vi "in_ensure monotonic.vi"(8 "X is monotonic":bool, 10 "Y":dbl[](array[numeric]), 11 "X":dbl[](array[numeric])) -> (2 "Y out":dbl[](array[numeric]), 3 "X out":dbl[](array[numeric]))   [LabVIEW 2010, in "NI_Gmath.lvlib"]
uses:
  NI_Gmath.lvlib
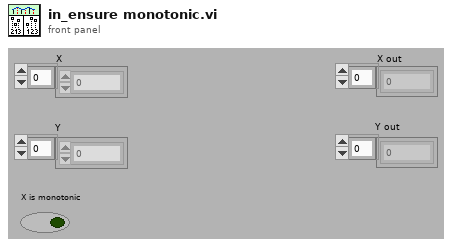
[diagram p1: front panel]
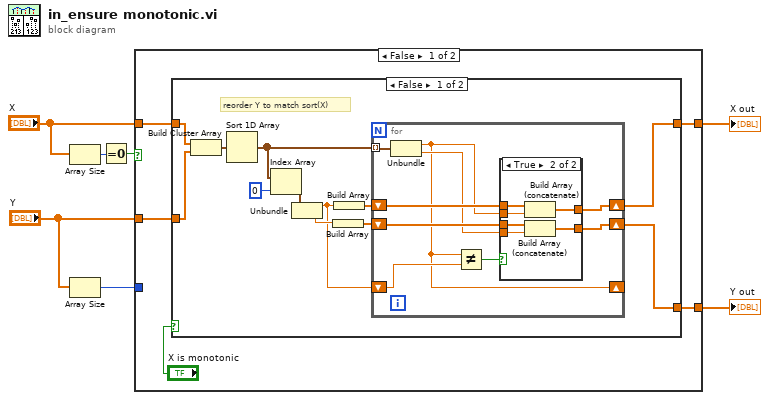
[diagram p0: block diagram]
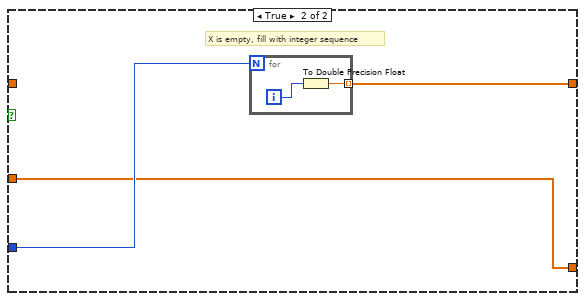
[diagram p4: hidden frame]
diagram:
  n1 = Array Size(array="X") -> (size(s)=w7:i32)
  n2 = Array Size(array="Y") -> (size(s)=w6:i32)
  n3 = Equal To 0?(x=w7) -> (x = 0?=w5:bool)
  n4 = case shown="False" w5 {
    tunnel: w6 -> [_ w46]
    tunnel: [w10 w44] -> w2
    tunnel: "X" -> [w12 _]
    tunnel: [w9 w45] -> w3
    tunnel: "Y" -> [w11 w44]
    frame False {
      n5 = case shown="False" "X is monotonic" {
        tunnel: w12 -> [w23 w42]
        tunnel: w11 -> [w22 w43]
        tunnel: [w13 w43] -> w10
        tunnel: [w14 w42] -> w9
        frame False {
          # "reorder Y to match sort(X)"
          n6 = Build Cluster Array(w23, w22) -> (w24:cluster{"Numeric":dbl, "Numeric":dbl}[])
          n7 = Sort 1D Array(array=w24) -> (sorted array=w21:cluster{"Numeric":dbl, "Numeric":dbl}[])
          n8 = Index Array(array=w21, index=0) -> (element=w19:cluster{"Numeric":dbl, "Numeric":dbl})
          n9 = Unbundle(w19) -> ("Numeric"=w15:dbl, "Numeric"=w18:dbl)
          n10 = Build Array(w18) -> (w17:dbl[])
          n11 = Build Array(w15) -> (w16:dbl[])
          n12 = for {
            tunnel: w21 -> [w33] mode=indexing
            shift-right: [w29] -> w14
            shift-left: w16 -> [w32]
            shift-right: [w28] -> w13
            shift-left: w17 -> [w31]
            shift-right: [w26] -> _
            shift-left: w15 -> [w27]
            n13 = Unbundle(w33) -> ("Numeric"=w26:dbl, "Numeric"=w30:dbl)
            n14 = Not Equal?(x=w26, y=w27) -> (x != y?=w25:bool)
            n15 = case shown="True" w25 {
              tunnel: w32 -> [w35 w41]
              tunnel: w31 -> [w34 w40]
              tunnel: w26 -> [_ w39]
              tunnel: w30 -> [_ w38]
              tunnel: [w35 w37] -> w29
              tunnel: [w34 w36] -> w28
              frame False {
              }
              frame True {
                n16 = Build Array (concatenate)(w41, w39) -> (w37:dbl[])
                n17 = Build Array (concatenate)(w40, w38) -> (w36:dbl[])
              }
            }
          }
        }
        frame True {
        }
      }
    }
    frame True {
      # "X is empty, fill with integer sequence"
      n18 = for {
        N: w46 -> [_]
        tunnel: [w47] -> w45 mode=indexing
        i -> [w48]
        n19 = To Double Precision Float(number=w48) -> (double precision float=w47:dbl)
      }
    }
  }
  "X out" <- w3
  "Y out" <- w2
